vi "OSICS_Write_and_Read.vi"(7 "Timeout (s)":sgl=60.0, 8 "error in (no error)":errorcluster, 10 "String to Send":string="*idn?", 11 "VISA IN":refnum<visa-resource-name>="COM3") -> (0 "error out":errorcluster, 2 "Message Available":string, 3 "VISA OUT":refnum<visa-resource-name>, 5 "ERR":i32)   [LabVIEW 2014, in "OSICS_LIB.lvlib"]
doc: "This Vi sends strings (Commands/Queries) to the OSICS module and wait for the operation to complete. In case a message is available, it is displayed. In case an error occured, it is displayed in ERR.\nError codes:\n-1210: Execution error\n-1331: Command Error\n-1332: TIMO - Time Out\n-1410: Device dependent error\n\nThis VI recognizes if the communication is established via RS232 or GPIB and applies the corresponding communication VI."
uses:
  OSICS_LIB.lvlib
  <vilib>/regexp/Match Regular Expression.xnode
  <vilib>/Instr/_visa.llb/VISA Configure Serial Port (Instr).vi
panel:
  # "Basic function to write/read commands/responses from\nOSICS mainframe and corresponding modules and\nother instruments"
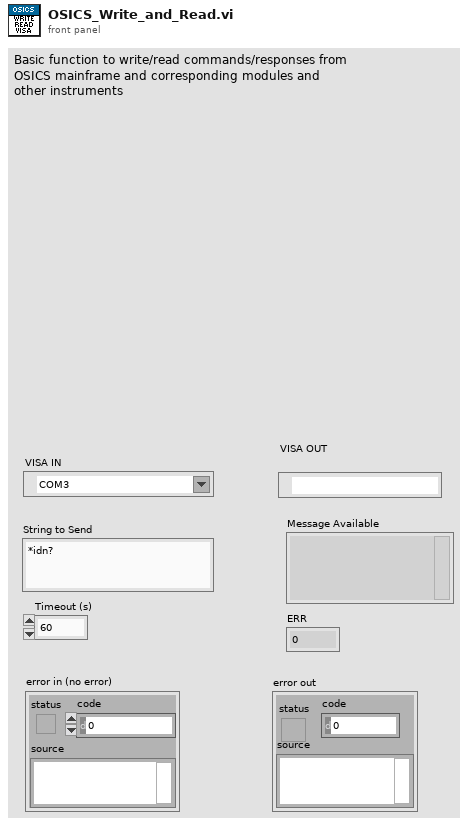
[diagram p1: front panel]
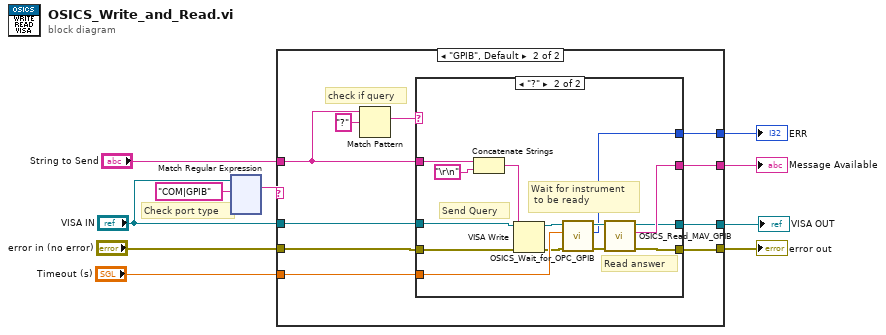
[diagram p0: block diagram]
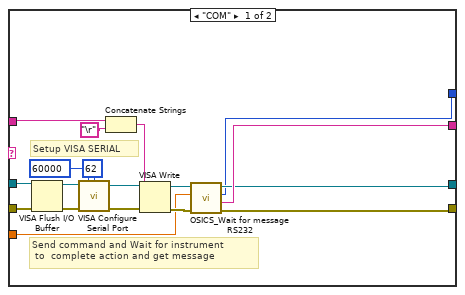
[diagram p2: hidden frame]
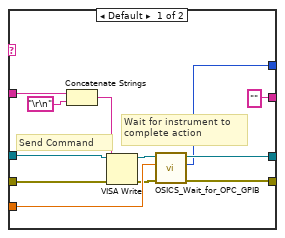
[diagram p3: hidden frame]
diagram:
  # "Check port type"
  n1 = xnode "Match Regular Expression"("input string"="VISA IN", "regular expression"="COM|GPIB") -> ("whole match"=w2:string)  [unwired: 4 in, 4 out]
  n2 = case shown="\"GPIB\", Default" w2 {
    tunnel: [w28 w38] -> w10
    tunnel: [w23 w37] -> w9
    tunnel: [w22 w36] -> w8
    tunnel: "Timeout (s)" -> [w16 w35]
    tunnel: "String to Send" -> [w27 w34]
    tunnel: "VISA IN" -> [w15 w31]
    tunnel: "error in (no error)" -> [w13 w30]
    tunnel: [w21 w29] -> w4
    frame "COM" {
      # "Setup VISA SERIAL"
      # "Send command and Wait for instrument\n to  complete action and get message"
      n3 = VISA Flush I/O Buffer(VISA resource name=w15, error in (no error)=w13) -> (VISA resource name out=w14:refnum<visa-resource-name>, error out=w12:errorcluster)  [unwired: 1 in]
      n4 = call-poly "VISA Configure Serial Port"("VISA resource name"=w14, "timeout (10sec)"=u32 60000, "termination char\n(0xA = '\\n' = LF)"=u8 62 ("termination char\n(0xA = '\\n' = LF)"), "error in (no error)"=w12) -> ("VISA resource name out"=w19:refnum<visa-resource-name>, "error out"=w17:errorcluster)  [unwired: 10 in]
      n5 = Concatenate Strings(w27, "\r") -> (w26:string)
      n6 = VISA Write(VISA resource name=w19, write buffer=w26, error in (no error)=w17) -> (VISA resource name out=w25:refnum<visa-resource-name>, error out=w24:errorcluster)  [unwired: 1 out]
      n7 = call "OSICS_Wait for message RS232.vi"("error in"=w24, "Timeout (s)"=w16, "VISA IN"=w25) -> ("error out"=w22:errorcluster, "Returned Message"=w28:string, "ERR"=w21:i32, "VISA OUT"=w23:refnum<visa-resource-name>)  [unwired: 5 in]
    }
    frame "GPIB", Default {
      # "check if query"
      n8 = Match Pattern(string=w34, regular expression="?") -> (match substring=w32:string)  [unwired: 1 in, 3 out]
      n9 = case shown="\"?\"" w32 {
        tunnel: w34 -> [w50 w64]
        tunnel: ["" ("Message") w59] -> w38
        tunnel: [w42 w58] -> w37
        tunnel: [w41 w57] -> w36
        tunnel: w31 -> [w47 w56]
        tunnel: w35 -> [w46 w55]
        tunnel: w30 -> [w45 w54]
        tunnel: [w39 w51] -> w29
        frame Default {
          # "Wait for instrument to\ncomplete action"
          # "Send Command"
          n10 = Concatenate Strings(w50, "\r\n") -> (w48:string)
          n11 = VISA Write(VISA resource name=w47, write buffer=w48, error in (no error)=w45) -> (VISA resource name out=w44:refnum<visa-resource-name>, error out=w43:errorcluster)  [unwired: 1 out]
          n12 = call "OSICS_Wait_for_OPC_GPIB.vi"("error in"=w43, "Timeout (s)"=w46, "VISA IN"=w44) -> ("error out"=w41:errorcluster, "ERR"=w39:i32, "VISA OUT"=w42:refnum<visa-resource-name>)  [unwired: 6 in]
        }
        frame "?" {
          # "Wait for instrument\n to be ready"
          # "Read answer"
          # "Send Query"
          n13 = Concatenate Strings(w64, "\r\n") -> (w62:string)
          n14 = VISA Write(VISA resource name=w56, write buffer=w62, error in (no error)=w54) -> (VISA resource name out=w53:refnum<visa-resource-name>, error out=w52:errorcluster)  [unwired: 1 out]
          n15 = call "OSICS_Wait_for_OPC_GPIB.vi"("error in"=w52, "Timeout (s)"=w55, "VISA IN"=w53) -> ("error out"=w60:errorcluster, "ERR"=w51:i32, "VISA OUT"=w61:refnum<visa-resource-name>)  [unwired: 6 in]
          n16 = call "OSICS_Read_MAV_GPIB.vi"("error in"=w60, "VISA IN"=w61) -> ("error out"=w57:errorcluster, "Message"=w59:string, "VISA OUT"=w58:refnum<visa-resource-name>)  [unwired: 7 in]
        }
      }
    }
  }
  "error out" <- w8
  "Message Available" <- w10
  "VISA OUT" <- w9
  "ERR" <- w4
